vi "get dependency list.vi"(8 "error in":errorcluster, 11 "Targets in":refnum<class "Targets.lvclass">) -> (0 "error out":errorcluster, 2 "files":T1[](array[typedef]), 3 "Targets out":refnum<class "Targets.lvclass">)   [LabVIEW 2013, in "PL Framework Configuration Tool.lvlib" / "Targets.lvclass"]
uses:
  Targets.lvclass
  TBM Configuration Node/deployment configuration.ctl
  Targets.lvclass/Targets.ctl
  TBM Configuration Node/TBM Configuration Node.lvclass
  Framework Configuration Classes/target configuration/PL_Target Configuration.lvclass/PL_Target Configuration.ctl
  Read additional files.vi
  Framework Configuration Classes/target configuration/Read load bitfile.vi
  Framework Configuration Classes/target configuration/Read bitfile path.vi
  read target configuration.vi
  Framework Configuration Classes/target configuration/PL_Target Configuration.lvclass
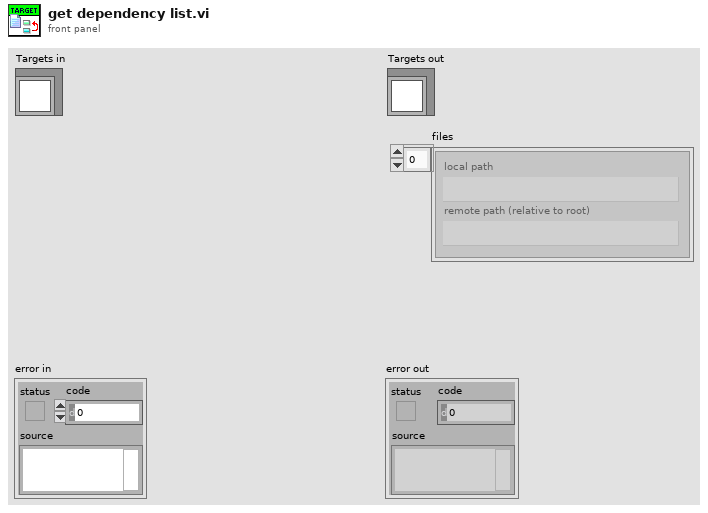
[diagram p1: front panel]
types:
  T1 = typedef "PL Framework Configuration Tool.lvlib/TBM Configuration Node.lvclass/deployment configuration.ctl" = cluster{"local path":path, "remote path (relative to root)":path}
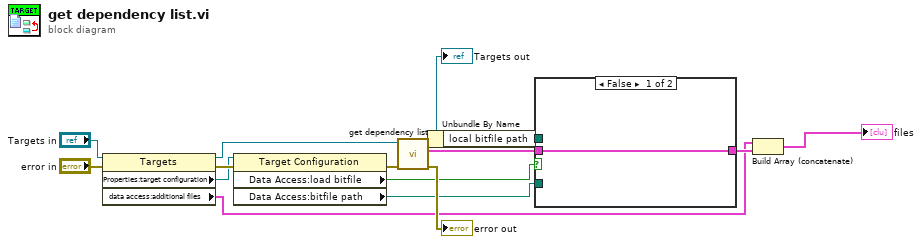
[diagram p0: block diagram]
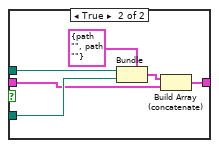
[diagram p2: hidden frame]
diagram:
  n1 = property class="Targets"(reference="Targets in", error in="error in") -> (reference out=w11:refnum<class "Targets.lvclass">, error out=w10:errorcluster, "Properties:target configuration"=w8:refnum<class "PL_Target Configuration.lvclass">, "data access:additional files"=w1:T1[])
  n2 = property class="Target Configuration"(reference=w8, error in=w10) -> (error out=w9:errorcluster, "Data Access:load bitfile"=w7:bool, "Data Access:bitfile path"=w4:path)  [unwired: 1 out]
  n3 = call-parent "get dependency list.vi"("error in"=w9, "TBM Configuration Node in"=w11) -> ("error out"=→"error out":errorcluster, "files"=w5:T1[], "TBM Configuration Node out"=w13:refnum<class "Targets.lvclass">)  [unwired: 7 in]
  "Targets out" <- w13
  n4 = Unbundle By Name(w13) -> ("local bitfile path"=w6:path)
  n5 = case shown="False" w7 {
    tunnel: w6 -> [_ w21]
    tunnel: w5 -> [w16 w18]
    tunnel: w4 -> [_ w20]
    tunnel: [w16 w17] -> w3
    frame False {
    }
    frame True {
      n6 = Bundle(cluster=T1 {"local path"=path "", "remote path (relative to root)"=path ""} ("deployment configuration"), "local path"=w21, "remote path (relative to root)"=w20) -> (w19:T1)
      n7 = Build Array (concatenate)(w19, w18) -> (w17:T1[])
    }
  }
  n8 = Build Array (concatenate)(w1, w3) -> (→"files":T1[])
